vi "ResultsDB Select Column Name List.vi"() -> (0 "error out":errorcluster, 3 "FirstRow":string[](array[string]))   [LabVIEW 2021, in "SQLite.lvclass"]
doc: "开始测试时根据条目自动创建条目条目，生产文件路径。\n#2020-6-8 13:25:45"
uses:
  SQLite.lvclass
  ProcutctionStatistic.ctl
  <userlib>/_OpenG.lib/array/array.llb/Search 1D Array (String)__ogtk.vi
  SQLite.lvclass/SQLite.ctl
  <userlib>/LabSQL/LabSQL.lvlib
  vi.lib_New/TopPath/TopPath.lvlib
  <userlib>/sushu/sushu.lvlib
panel:
  out "产量统计":T1
  out "CMD":string
  out "subarray":string[](array[string])
  out "number (0 to 1)":dbl
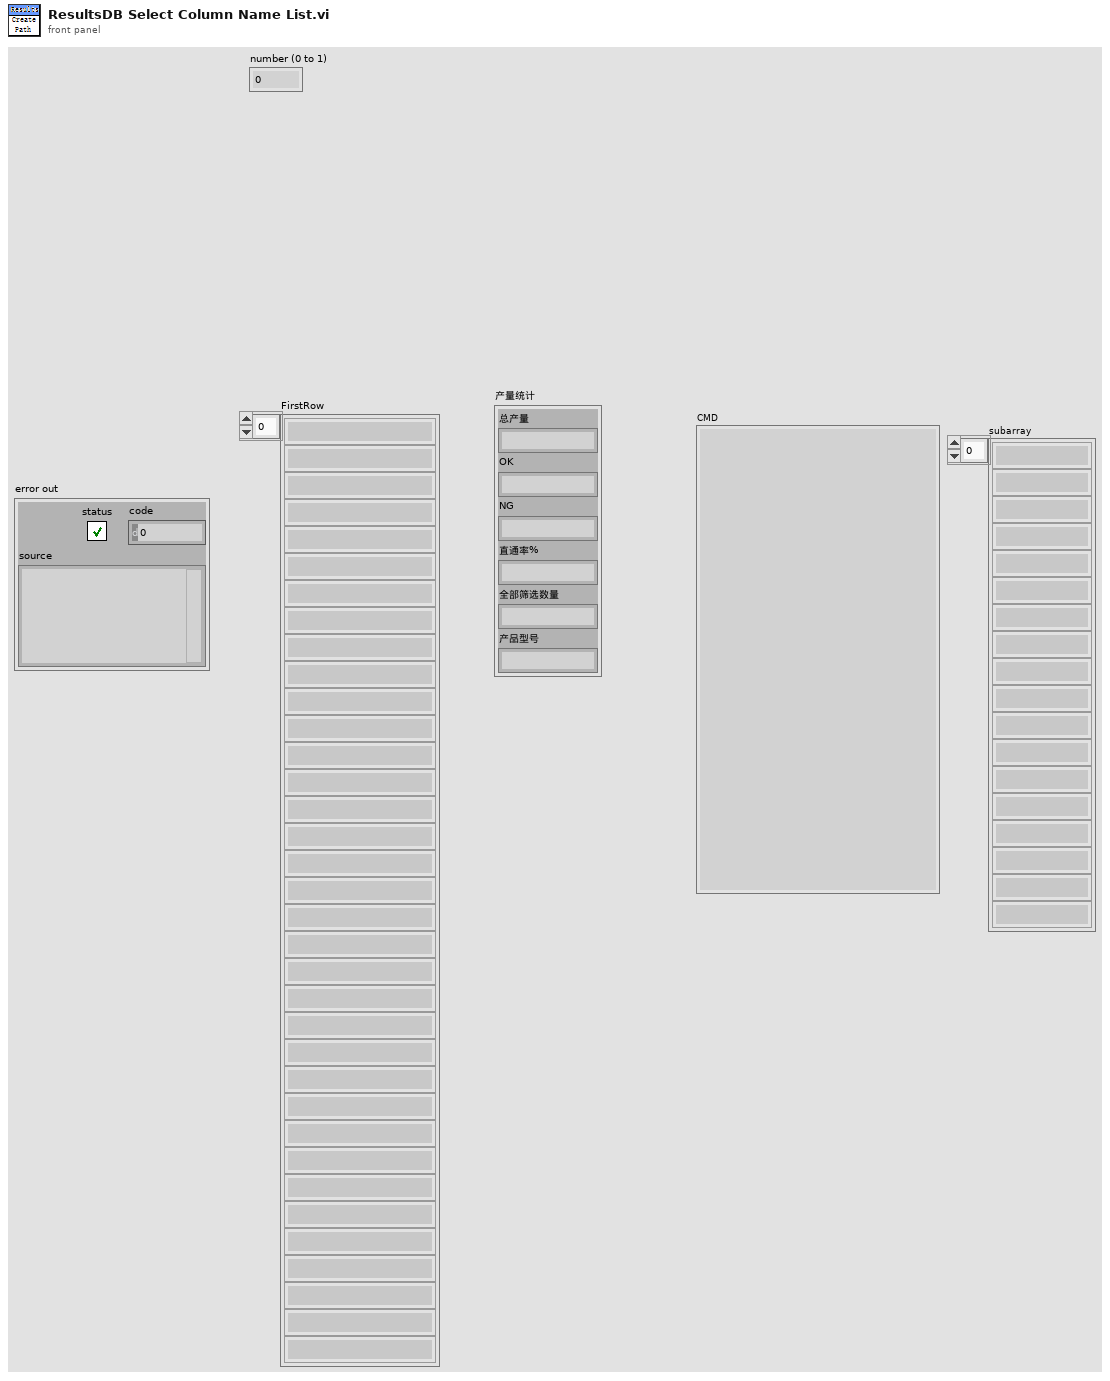
[diagram p1: front panel]
types:
  T1 = typedef "SQLite.lvclass/ProcutctionStatistic.ctl" = cluster{"总产量":string, "OK":string, "NG":string, "直通率%":string, "全部筛选数量":string, "产品型号":string}
  T2 = cluster{"Core":cluster{"Current VI Reference":refnum<vi>, "Close Panel on Exit?":bool}, "VI Name":string, "Row Numbers":string, "Update?":bool, "Results Folder path":path, "CMD":string, "RowNum":i32, "ResultFilePath":path, "InsertTimes":i32, "length":i32}
  T3 = enum16{"Other", "SQL2008", "SQLite", "Access", "MySQL"}
  T4 = typedef "TopPath.lvlib/Top Path.ctl" = cluster{"LV Source":path, "FilePath":path, "Data":path}
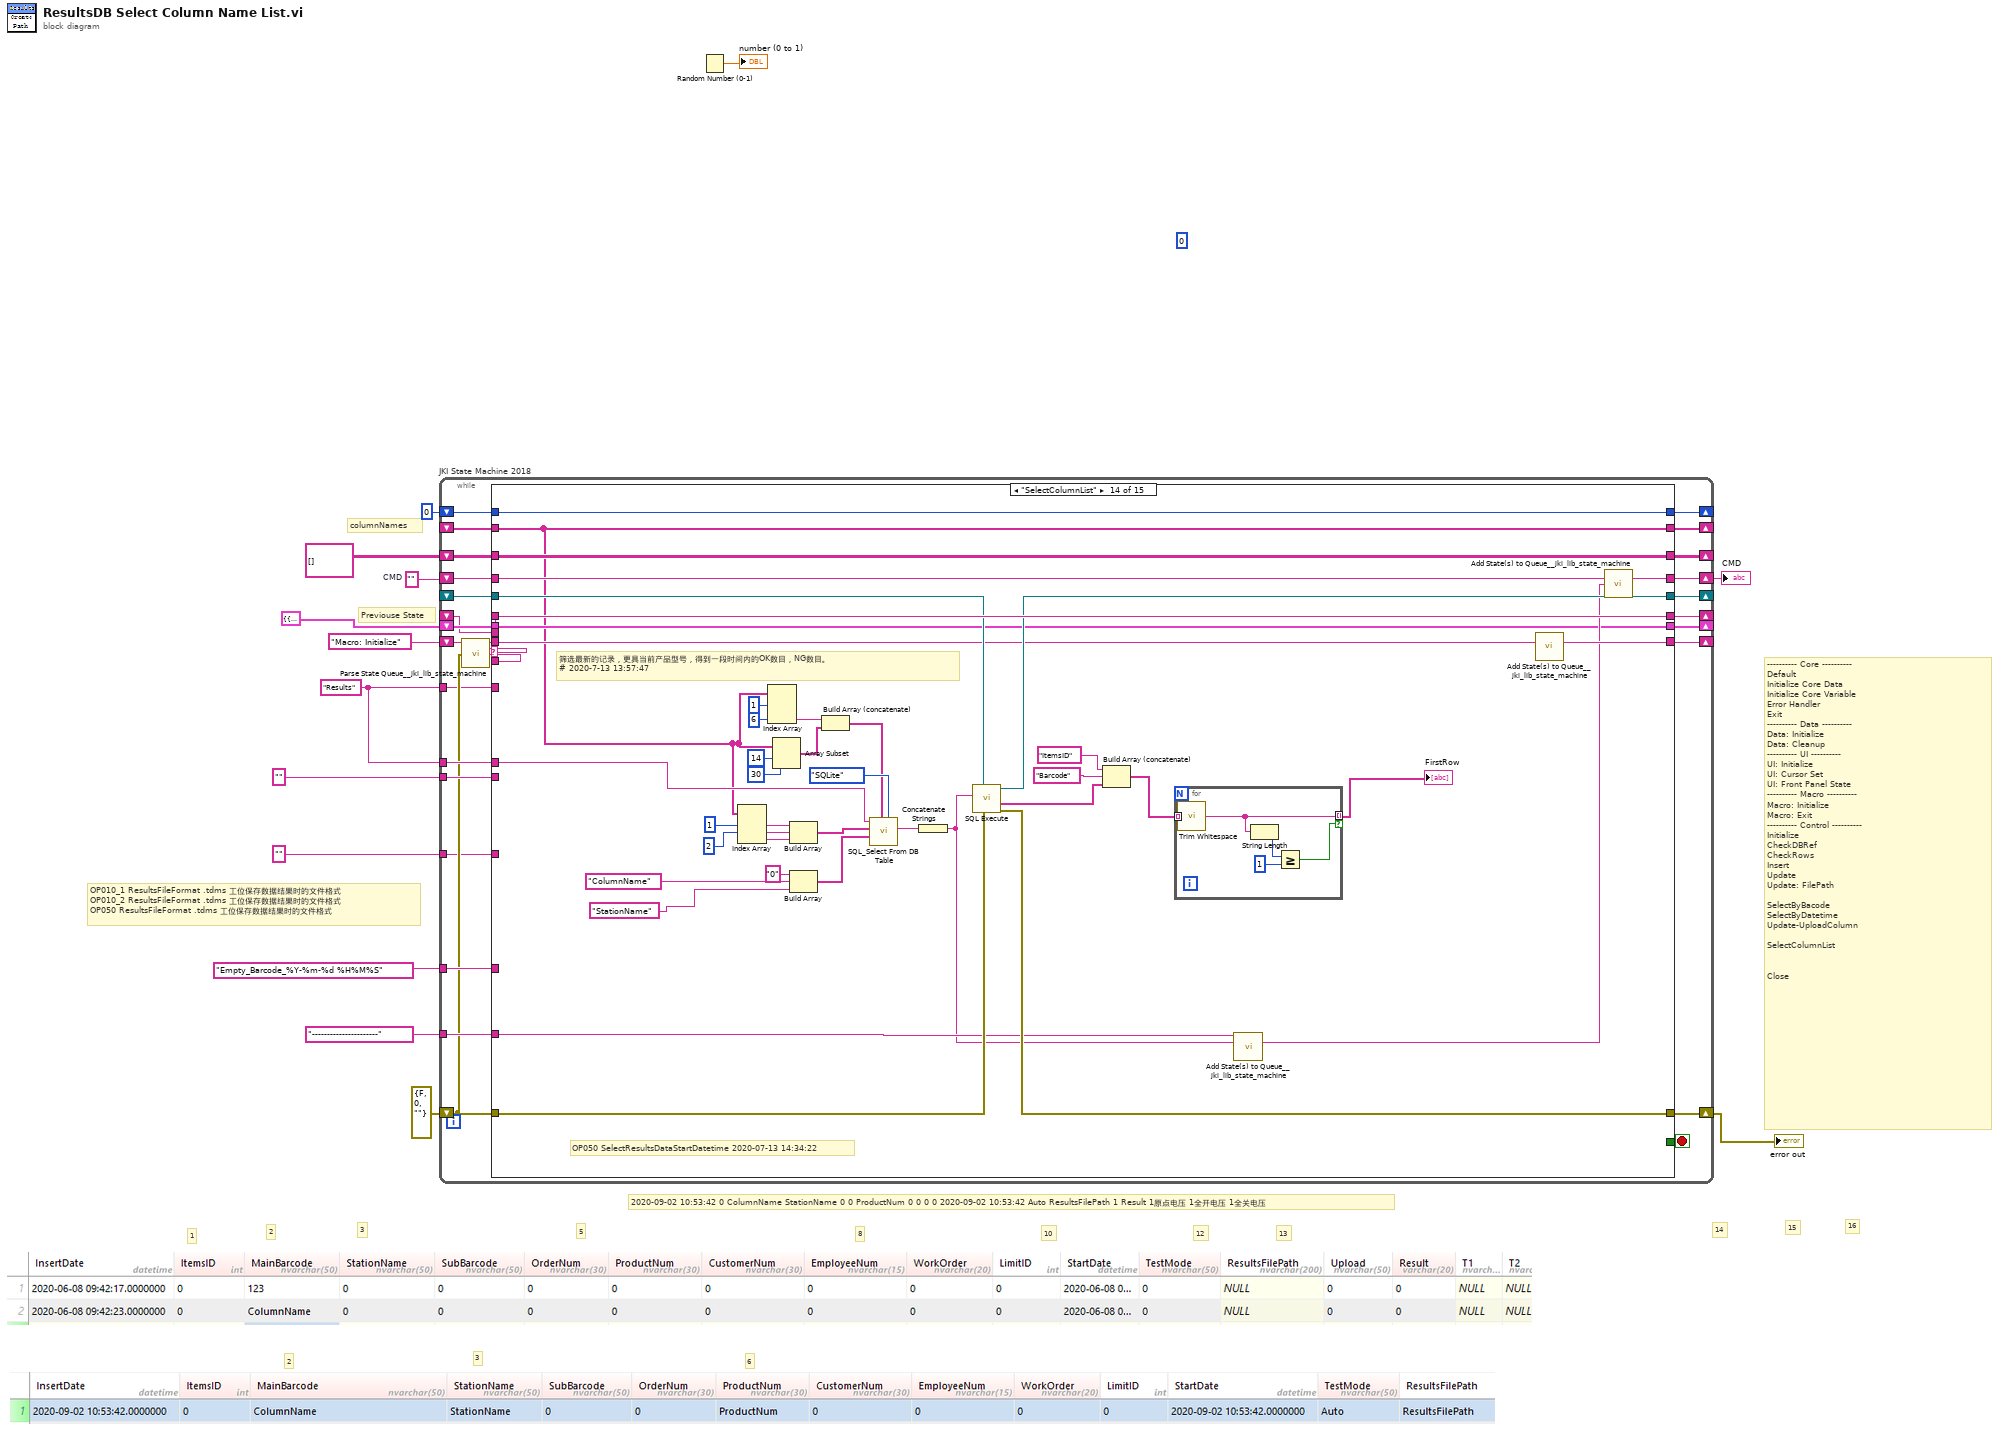
[diagram p0: block diagram]
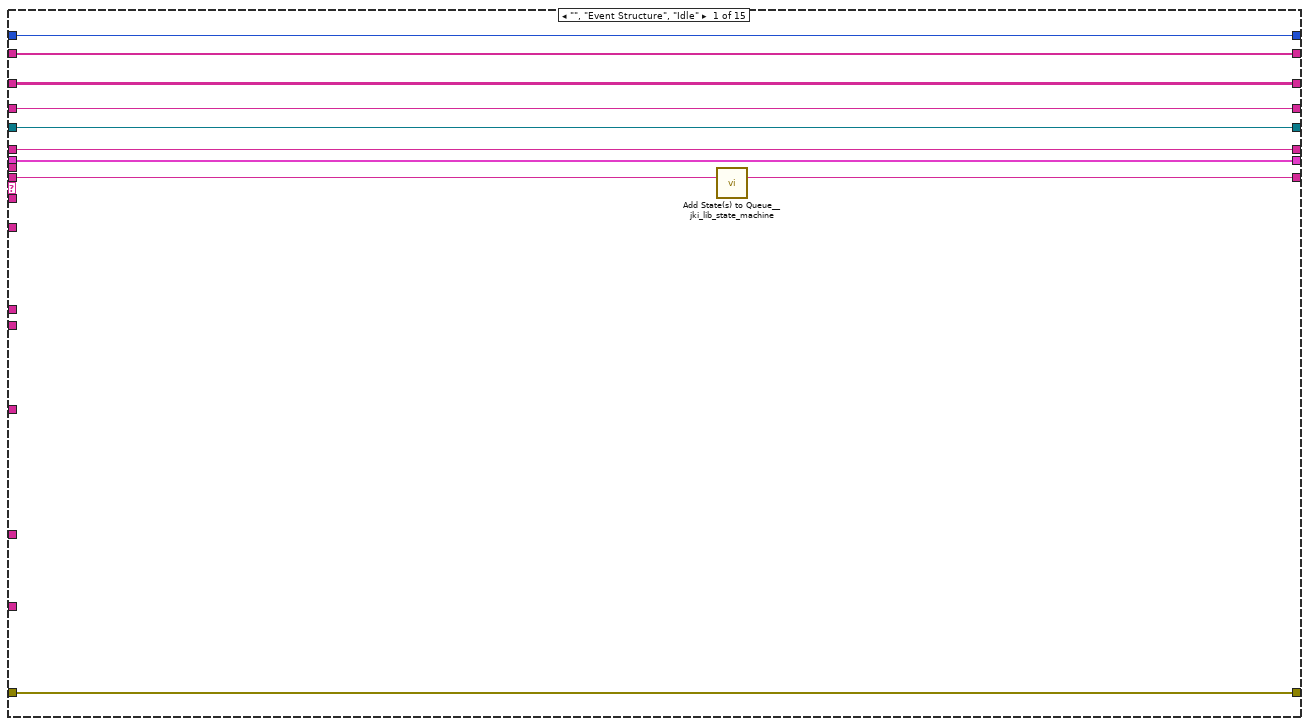
[diagram p2: hidden frame]
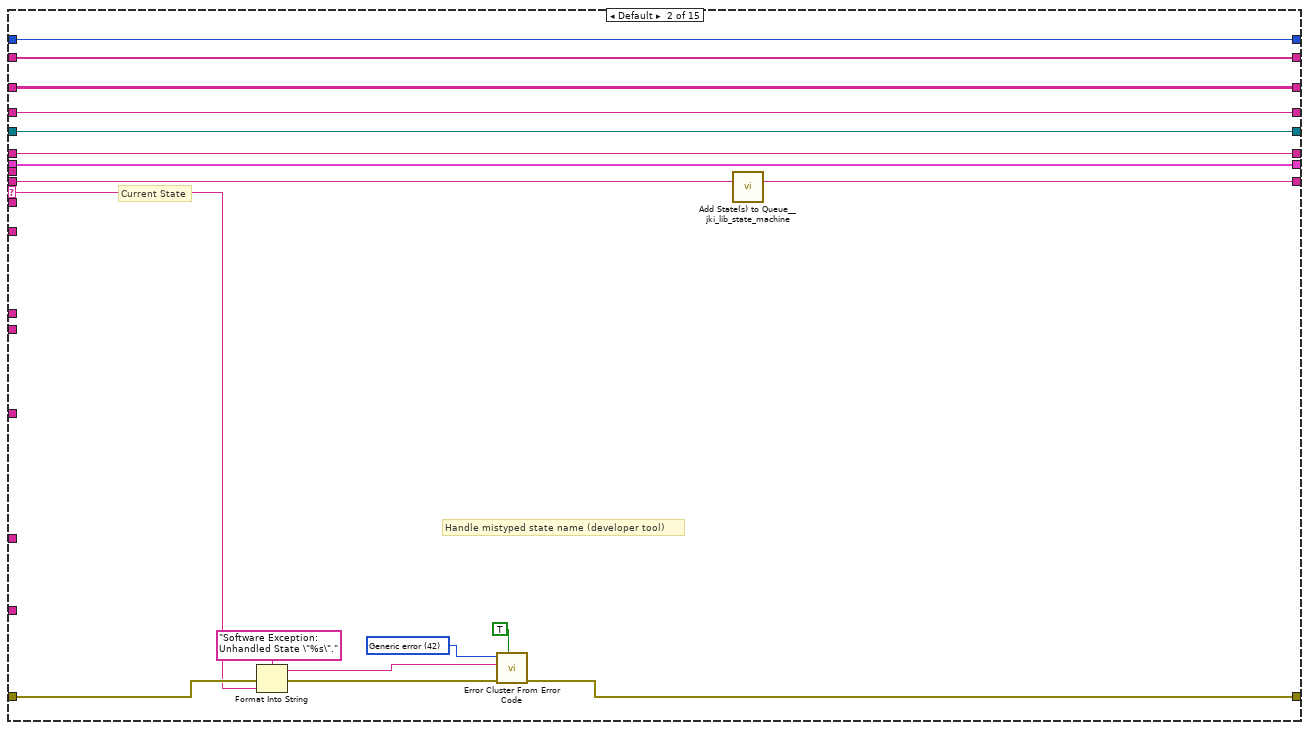
[diagram p3: hidden frame]
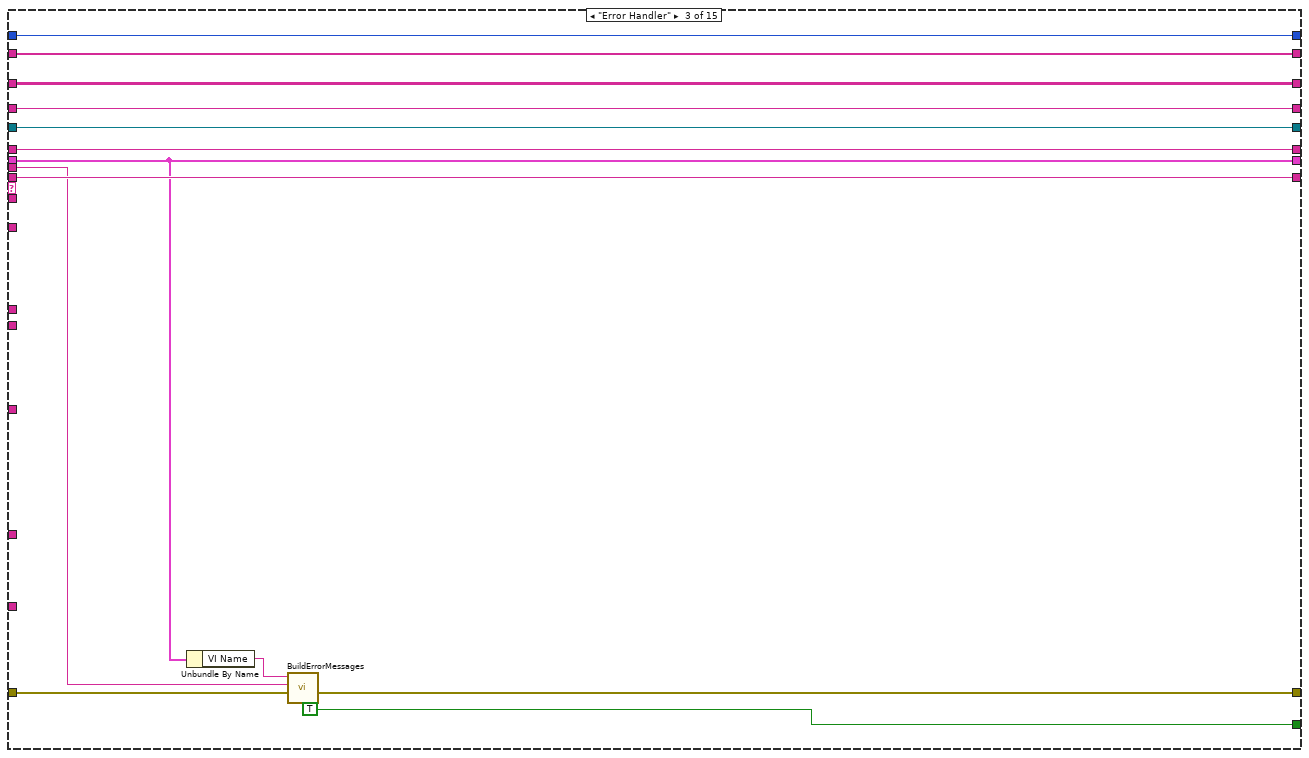
[diagram p4: hidden frame]
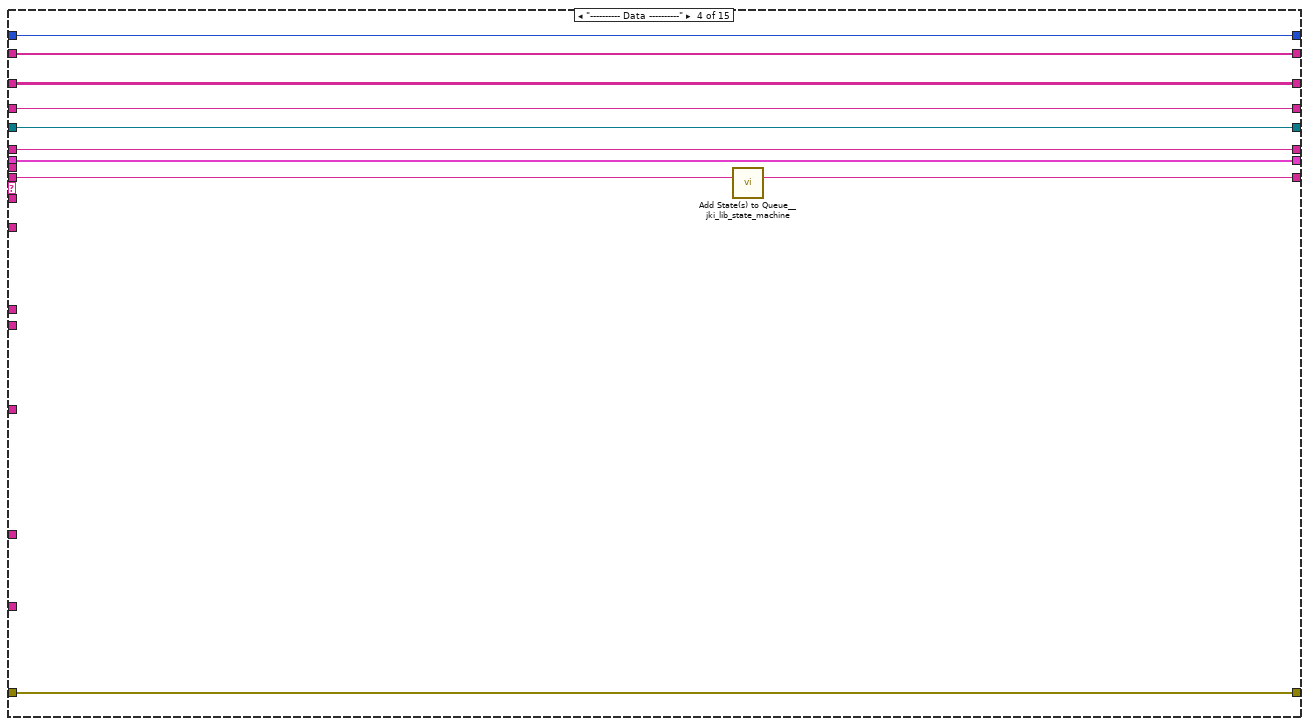
[diagram p5: hidden frame]
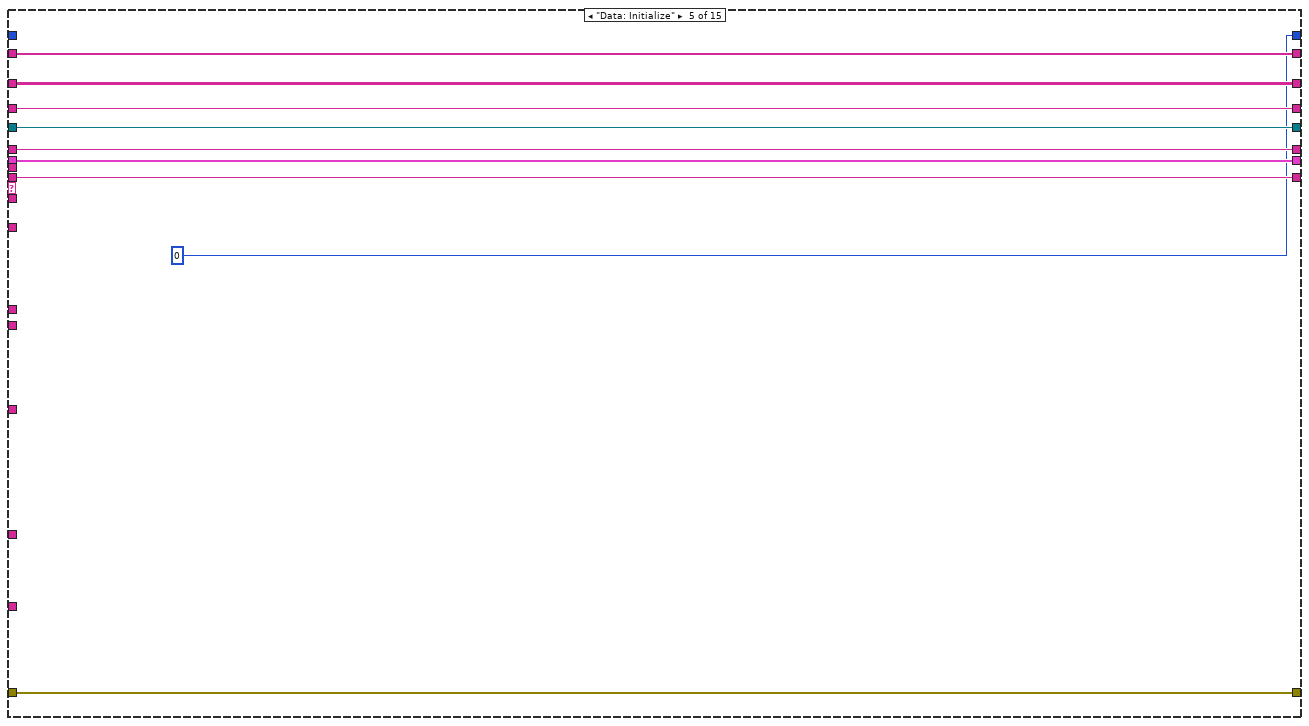
[diagram p6: hidden frame]
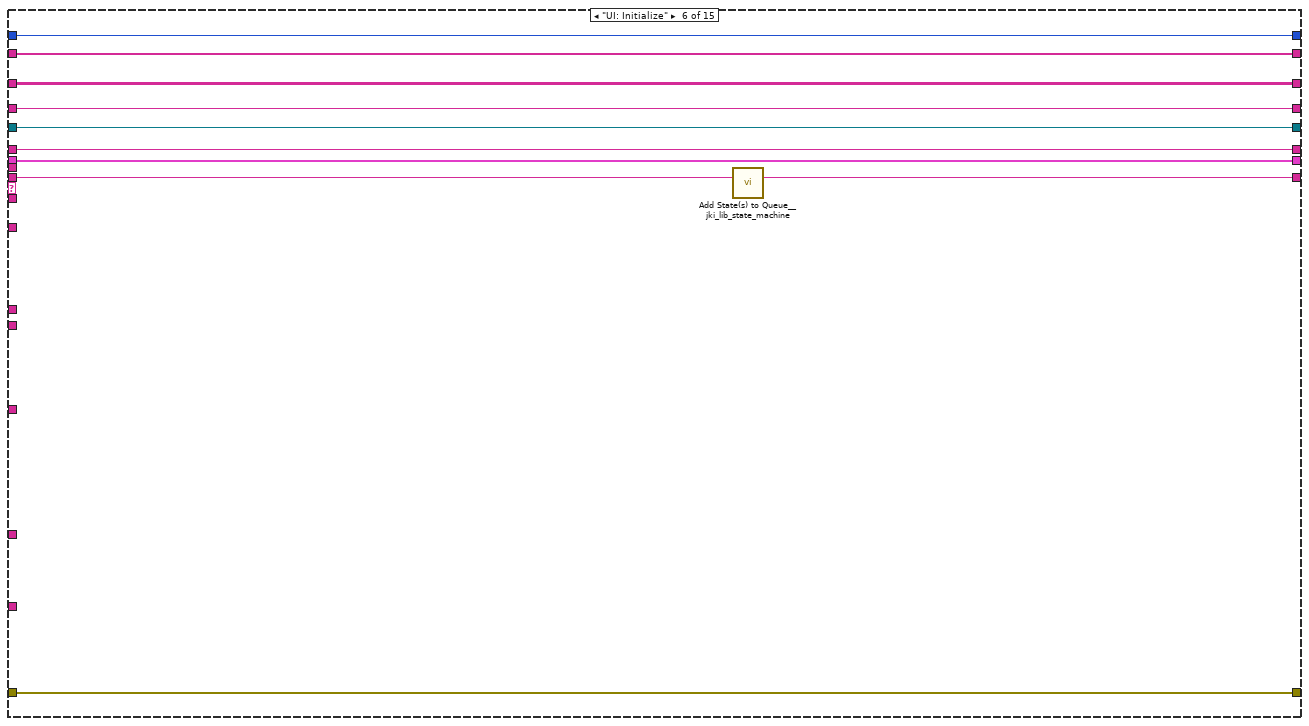
[diagram p7: hidden frame]
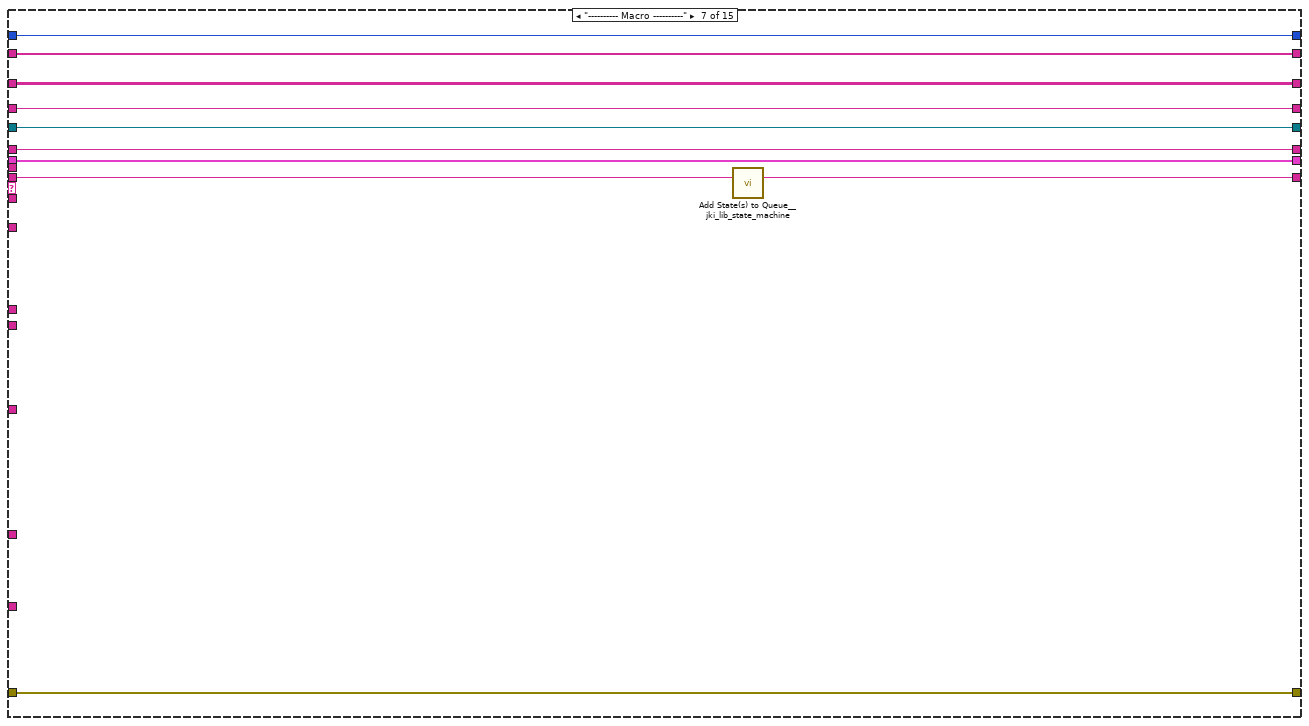
[diagram p8: hidden frame]
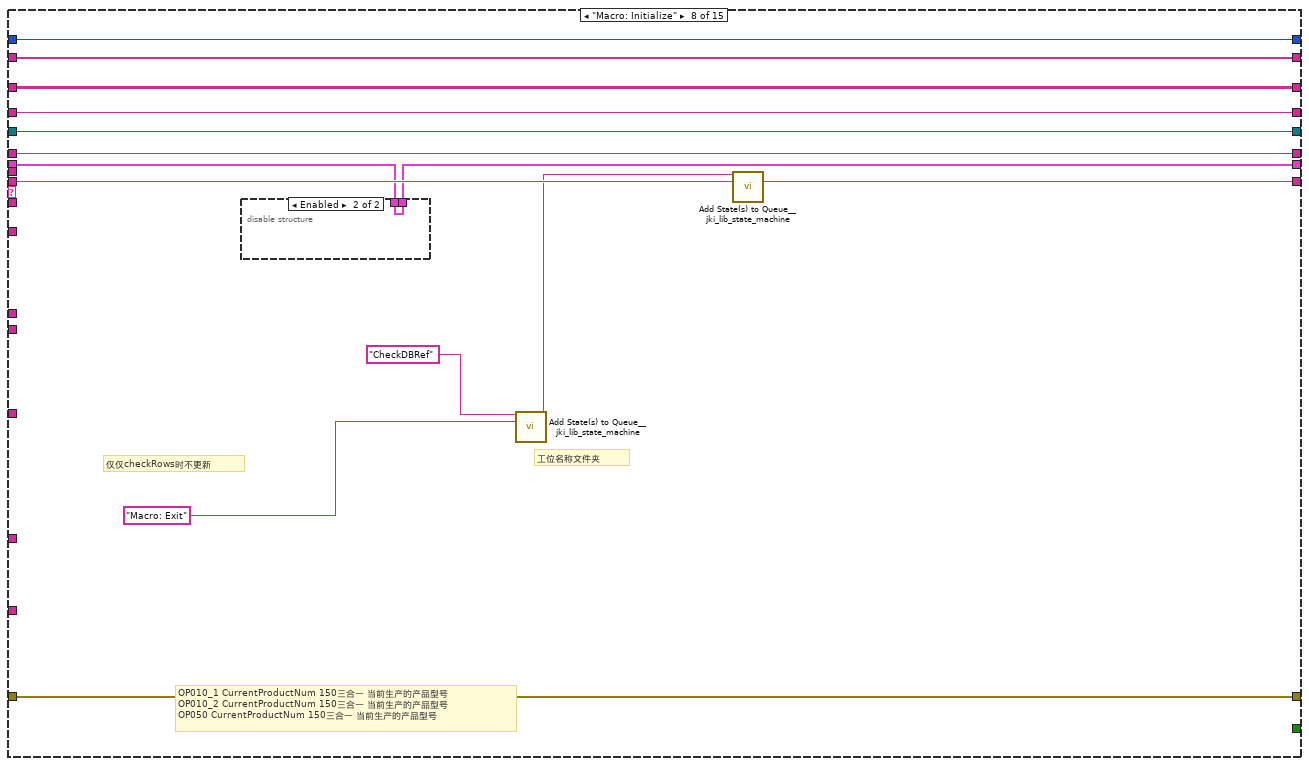
[diagram p9: hidden frame]
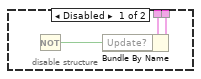
[diagram p10: hidden frame]
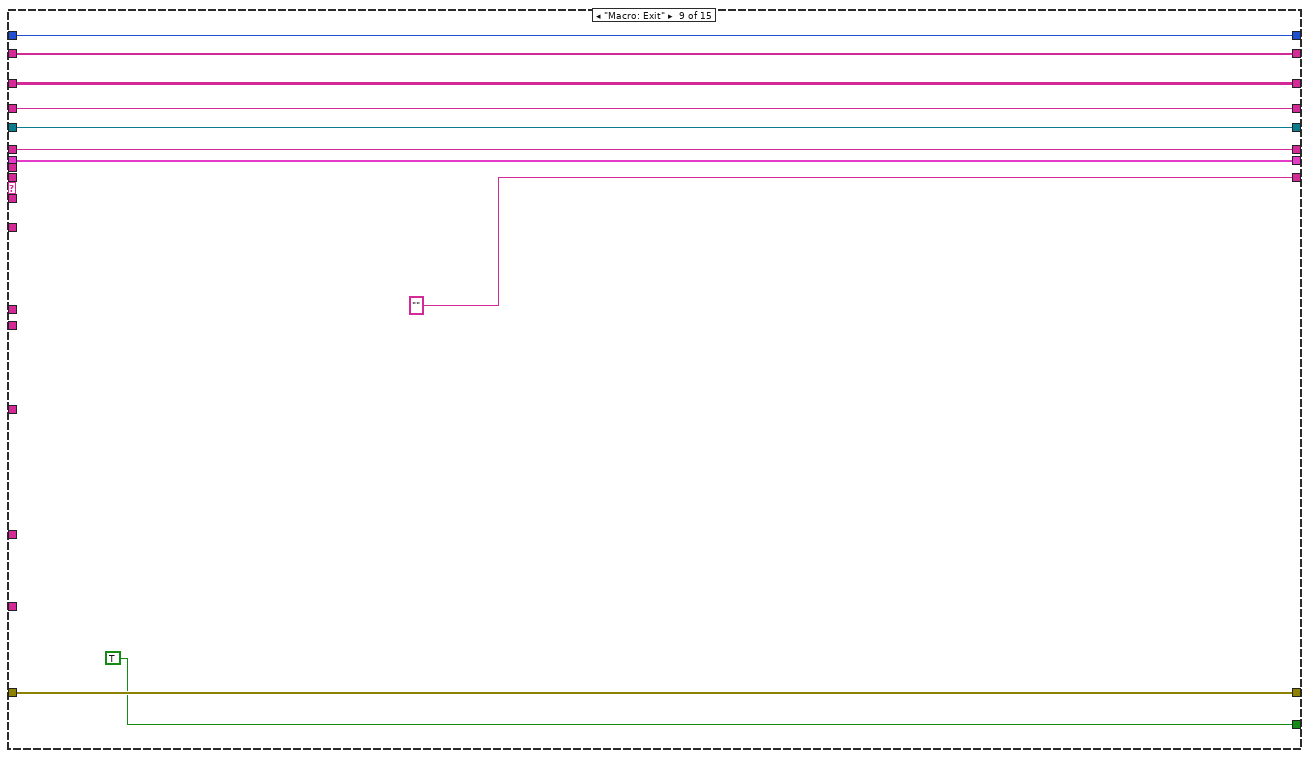
[diagram p11: hidden frame]
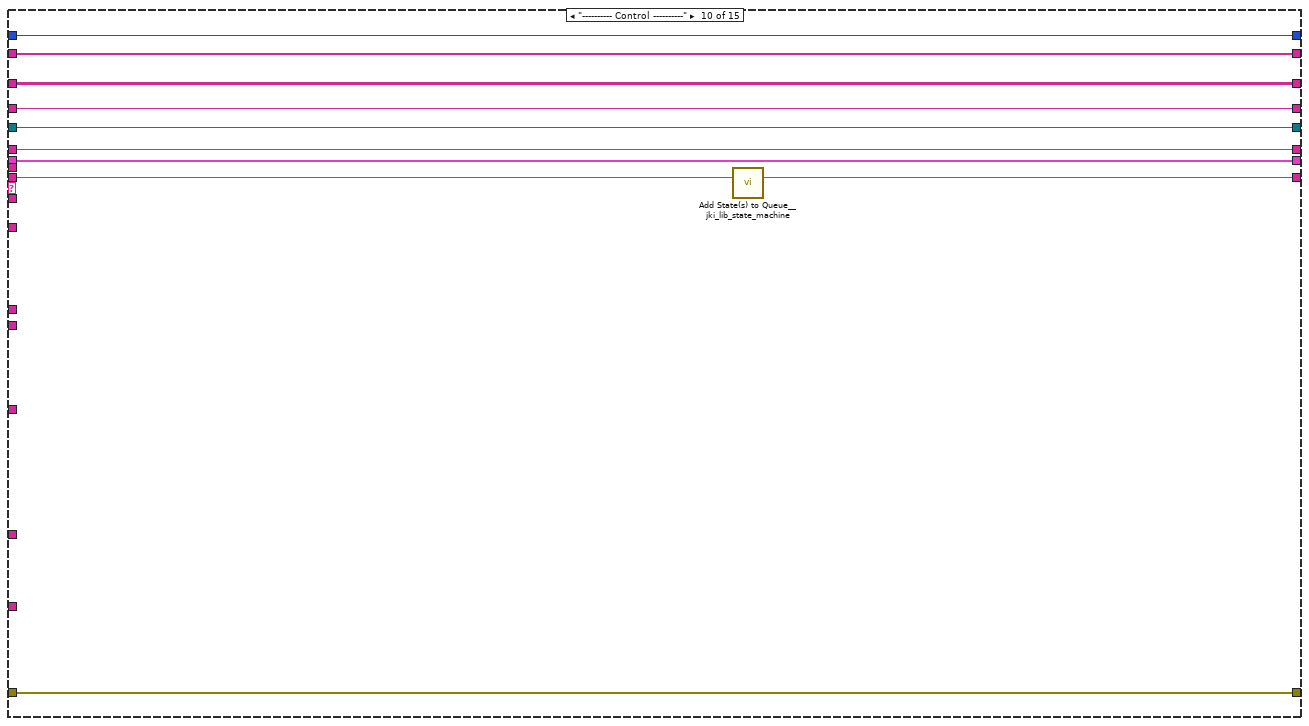
[diagram p12: hidden frame]
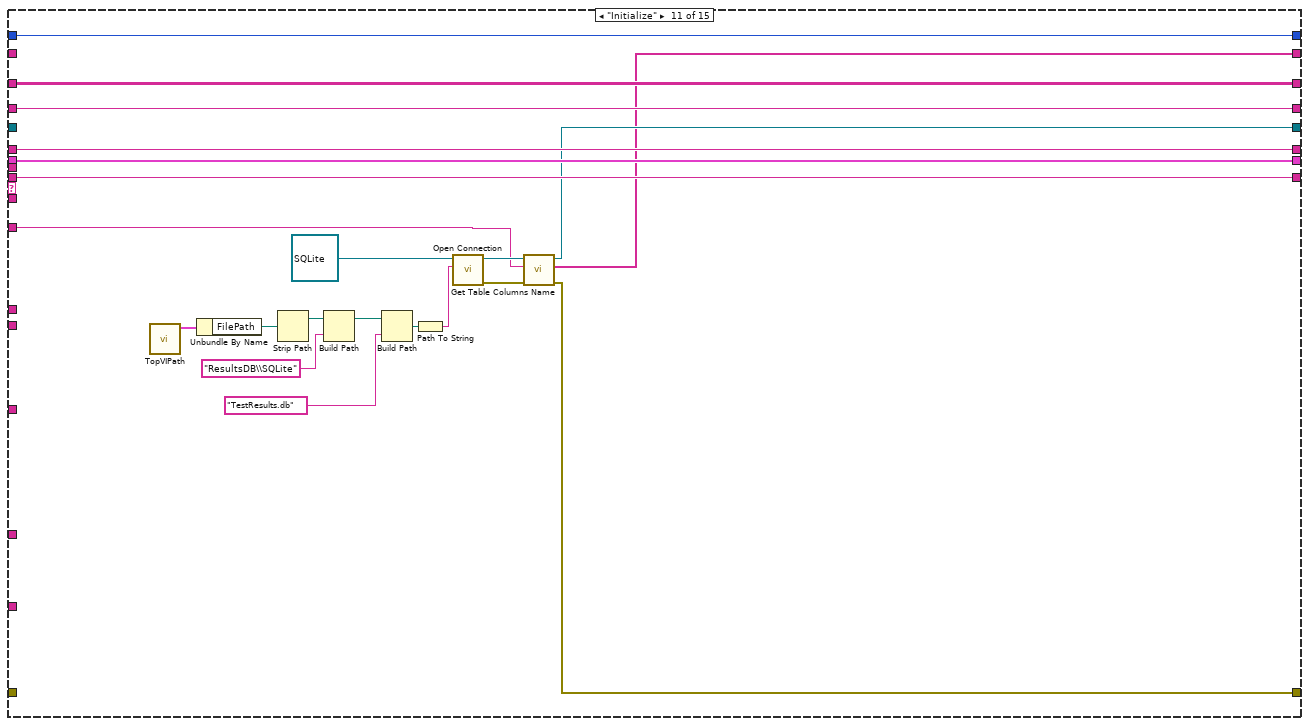
[diagram p13: hidden frame]
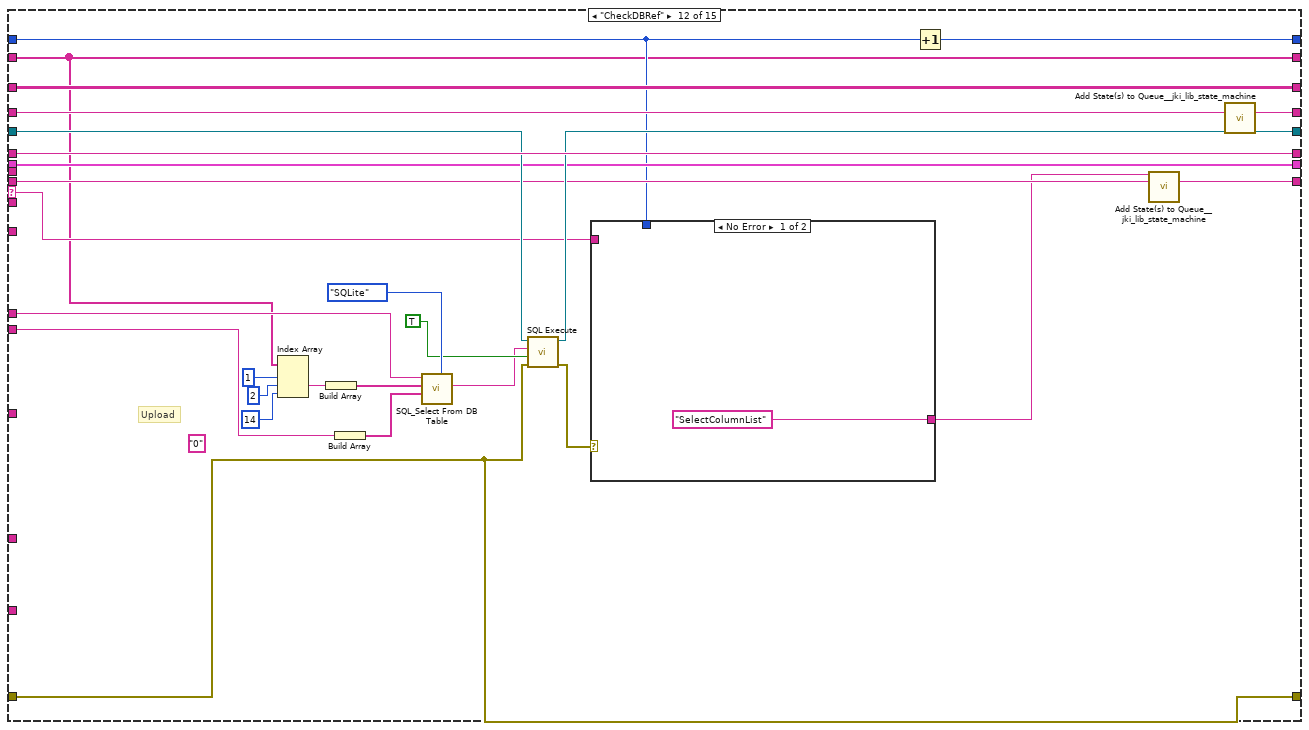
[diagram p14: hidden frame]
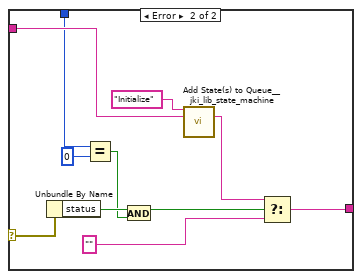
[diagram p15: hidden frame]
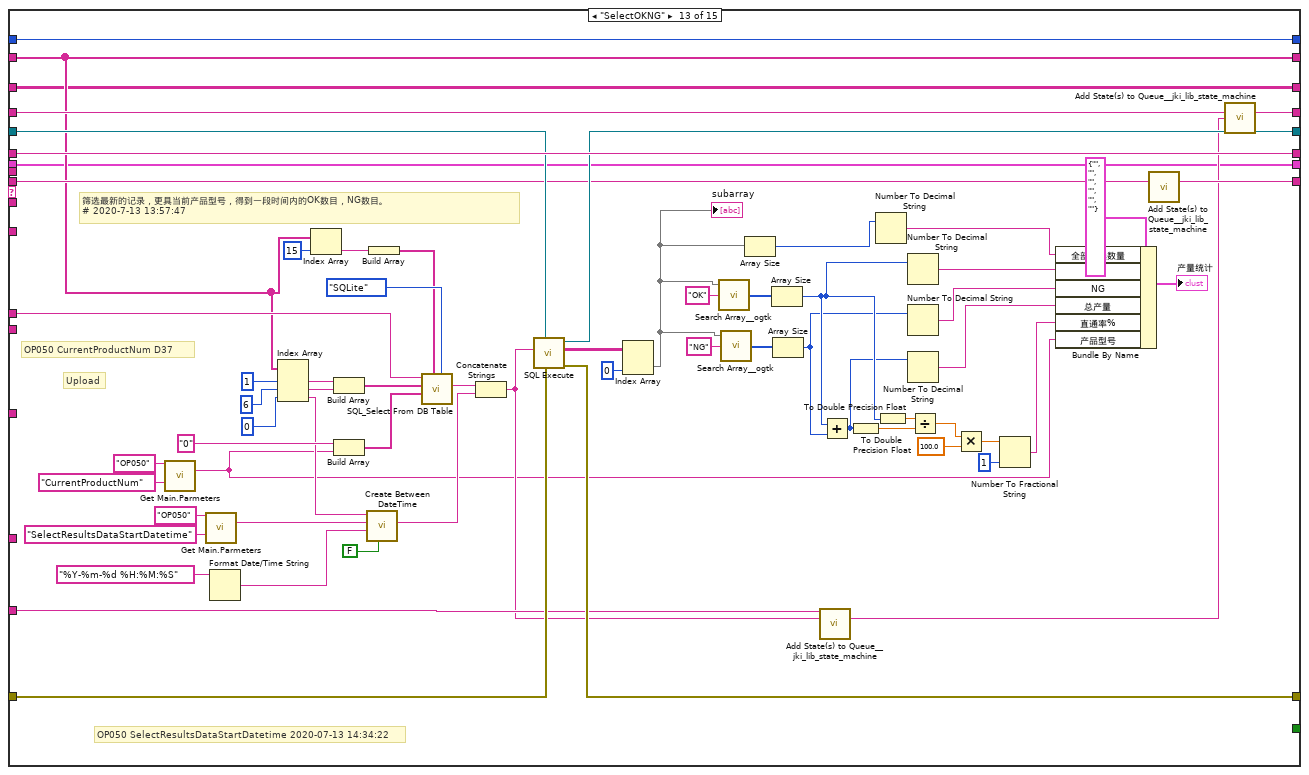
[diagram p16: hidden frame]
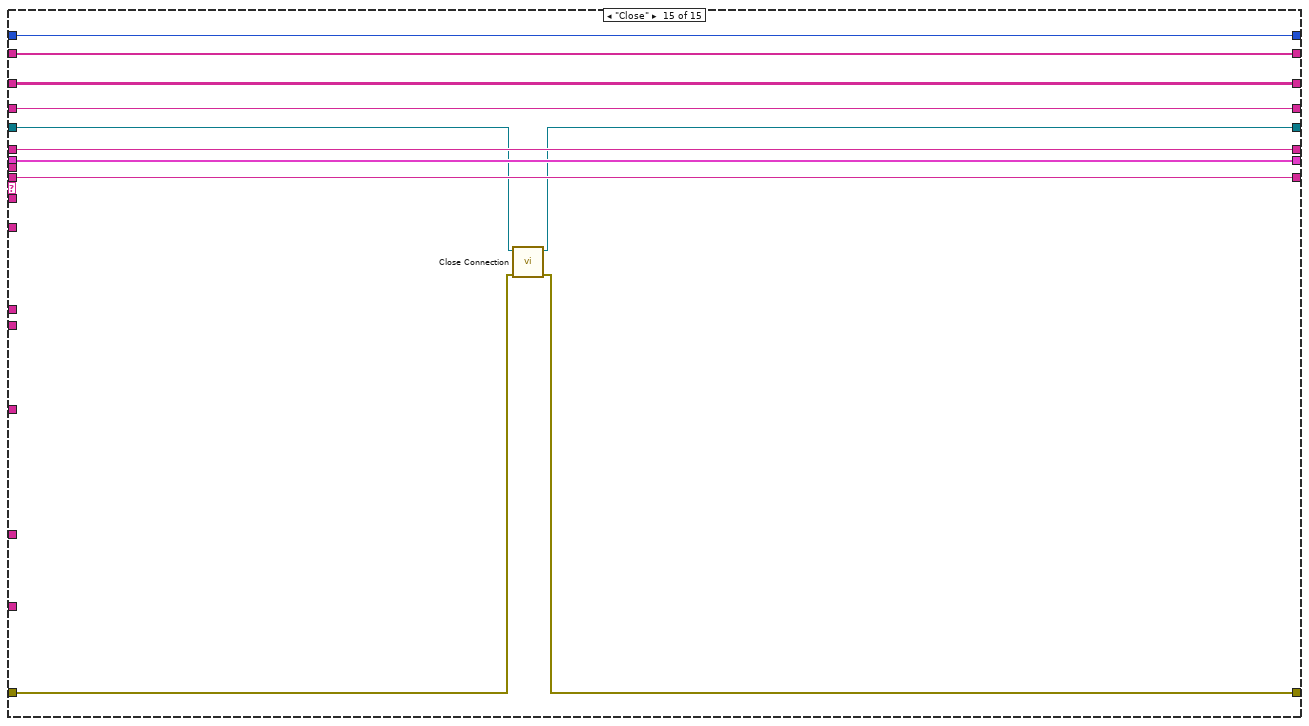
[diagram p17: hidden frame]
diagram:
  w5 = "Results" ("TableName")
  w7 = ""  # CMD
  (unwired) 0 ("index (row)")
  # "6"
  # "3"
  # "2"
  # "2020-09-02 10:53:42\t0\tColumnName\tStationName\t0\t0\tProductNum\t0\t0\t0\t0\t2020-09-02 10:53:42\tAuto\tResultsFilePath\t1\tResult\t1原点电压\t1全开电压\t1全关电压"
  # "columnNames"
  # "OP010_1\tResultsFileFormat\t.tdms\t工位保存数据结果时的文件格式\nOP010_2\tResultsFileFormat\t.tdms\t工位保存数据结果时的文件格式\nOP050\tResultsFileFormat\t.tdms\t工位保存数据结果时的文件格式"
  # "16"
  # "15"
  # "14"
  # "13"
  # "12"
  # "10"
  # "8"
  # "5"
  # "3"
  # "2"
  # "1"
  # "Previouse State"
  # "---------- Core ----------\nDefault\nInitialize Core Data\nInitialize Core Variable\nError Handler\nExit\n---------- Data ----------\nData: Initialize\nData: Cleanup\n---------- UI ----------\nUI: Initialize\nUI: Cursor Set\nUI: Front Panel State\n---------- Macro ----------\nMacro: Initialize\nMacro: Exit\n---------- Control ----------\nInitialize\nCheckDBRef\nCheckRows\nInsert\nUpdate\nUpdate: FilePath\n\nSelectByBacode\nSelectByDatetime\nUpdate-UploadColumn\n\nSelectColumnList\n\n\nClose"
  n1 = while "JKI State Machine 2018" {
    shift-right: [w36] -> _
    shift-left: T2 {"Core"={"Current VI Reference"=refnum, "Close Panel on Exit?"=FALSE}, "VI Name"="", "Row Numbers"="", "Update?"=FALSE, "Results Folder path"=path "", "CMD"="", "RowNum"=0, "ResultFilePath"=path "", "InsertTimes"=0, "length"=3} ("Data") -> [w35]
    shift-right: [w39] -> w2
    shift-left: errorcluster {"status"=FALSE, "code"=0, "source"=""} ("error out") -> [w21]
    shift-right: [w38] -> _
    shift-left: "Macro: Initialize" -> [w40]
    shift-right: [w33] -> _
    shift-left: _ -> [w34]
    shift-right: [w31] -> _
    shift-left: _ -> [w30]
    tunnel: "" ("MainBarcode") -> [w29]
    tunnel: w5 -> [w28]
    tunnel: "Empty_Barcode_%Y-%m-%d %H%M%S" ("time format string (%c)") -> [w27]
    shift-right: [w26] -> w1
    shift-left: w7 -> [w25]
    tunnel: "----------------------" ("State(s) in (\"\")") -> [w24]
    shift-right: [w22] -> _
    shift-left: string[][] [] ("Table Control") -> [w23]
    tunnel: "" ("ItemsID") -> [w20]
    tunnel: w5 -> [w19]
    shift-right: [w18] -> _
    shift-left: _ -> [w17]
    shift-right: [w15] -> _
    shift-left: 0 -> [w16]
    stop <- w37 stop-if-true
    n2 = call <vilib>:"Parse State Queue__jki_lib_state_machine.vi"("State Queue"=w40, "Error In (no error)"=w21) -> ("Remaining States"=w42:string, "Current State"=w32:string, "Arguments"=w41:string)  [unwired: 10 in, 1 out]
    n3 = case shown="\"SelectColumnList\"" w32 {
      selector: w32 -> [_ w59 _ _ _ _ _ _ _ _ _ w186 _ _ _]
      tunnel: w42 -> [w52 w63 w81 w92 w98 w111 w121 w135 _ w159 w180 w196 w274 w315 w341]
      tunnel: w41 -> [_ _ _ _ _ _ _ _ _ _ _ _ _ _ _]
      tunnel: w35 -> [w49 w61 w78 w89 w99 w109 w118 w130 w148 w156 w179 w192 w243 w299 w340]
      tunnel: [w50 w65 w74 w90 w101 w108 w119 w131 w149 w157 w163 w185 w272 w313 w331] -> w39
      tunnel: w21 -> [w50 w64 w75 w90 w101 w108 w119 w131 w149 w157 _ w185 w273 w314 w332]
      tunnel: [w51 w62 w81 w91 w98 w110 w120 w134 "" w158 w180 w197 w275 w316 w341] -> w38
      tunnel: [_ _ TRUE _ _ _ _ _ TRUE _ _ _ _ _ _] -> w37
      tunnel: [w49 w61 w78 w89 w99 w109 w118 w125 w148 w156 w179 w192 w243 w299 w340] -> w36
      tunnel: w34 -> [w48 w58 w80 w88 w100 w107 w117 w133 w147 w155 _ w200 w277 w318 w334]
      tunnel: [w48 w58 w80 w88 w100 w107 w117 w133 w147 w155 w164 w199 w276 w317 w333] -> w33
      tunnel: w32 -> [w47 w57 w79 w87 w97 w106 w116 w132 w145 w154 w178 w207 w284 w325 w339]
      tunnel: [w47 w57 w79 w87 w97 w106 w116 w132 w145 w154 w178 w207 w284 w325 w339] -> w31
      tunnel: w30 -> [_ _ w76 _ _ _ _ _ _ _ _ _ _ _ _]
      tunnel: w29 -> [_ _ _ _ _ _ _ _ _ _ _ w201 _ _ _]
      tunnel: w28 -> [_ _ _ _ _ _ _ _ _ _ _ w202 w278 w319 _]
      tunnel: w27 -> [_ _ _ _ _ _ _ _ _ _ _ _ _ _ _]
      tunnel: w25 -> [w46 w56 w73 w86 w96 w105 w115 w127 w143 w153 w177 w194 w270 w311 w338]
      tunnel: [w46 w56 w73 w86 w96 w105 w115 w127 w143 w153 w177 w195 w271 w312 w338] -> w26
      tunnel: w24 -> [_ _ _ _ _ _ _ _ _ _ _ _ w267 w308 _]
      tunnel: w23 -> [w45 w55 w72 w85 w95 w104 w114 w126 w142 w152 w176 w188 w246 w300 w337]
      tunnel: [w45 w55 w72 w85 w95 w104 w114 w126 w142 w152 w176 w188 w246 w300 w337] -> w22
      tunnel: w20 -> [_ _ _ _ _ _ _ _ _ _ _ _ _ _ _]
      tunnel: w19 -> [_ _ _ _ _ _ _ _ _ _ w162 _ _ _ _]
      tunnel: w17 -> [w44 w54 w71 w84 w94 w103 w113 w124 w141 w151 _ w181 w250 w298 w336]
      tunnel: [w44 w54 w71 w84 w94 w103 w113 w124 w141 w151 w161 w181 w250 w298 w336] -> w18
      tunnel: w16 -> [w43 w53 w70 w83 _ w102 w112 w122 w140 w150 w160 w182 w259 w304 w335]
      tunnel: [w43 w53 w70 w83 0 w102 w112 w122 w140 w150 w160 w183 w259 w304 w335] -> w15
      frame "", "Event Structure", "Idle" {
        n4 = call <vilib>:"Add State(s) to Queue__jki_lib_state_machine.vi"("State(s) in (\"\")"=w52) -> ("States Out"=w51:string)  [unwired: 14 in]
      }
      frame Default {
        w68 = 42 items=["No error", "Argument error", "Memory is full", "Out of zone", "End of file", "File already open", "Generic file I/O error", "File not found", "File permission error", "Disk is full", "Duplicate path", "Too many files open", "System feature not enabled", "Resource file not found", "Cannot add resource", "Resource not found", "Image not found", "Image memory error", "Pen does not exist", "Config type invalid", "Config token not found", "Config parse error", "Config memory error", "Bad external code format", "Bad external code offset", "External code not present", "Null window", "Destroy window error", "Null menu", "Print aborted", "Bad print record", "Print driver error", "Windows error during printing", "Memory error during printing", "Print dialog error", "Generic print error", "Invalid device refnum", "Device not found", "Device parameter error", "Device unit error", "Cannot open device", "Device call aborted", "Generic error", "Cancelled by user", "Object ID too low", "Object ID too high", "Object not in heap", "Unknown heap", "Unknown object (invalid DefProc)", "Unknown object (DefProc not in table)", "Message out of range", "Invalid (null) method", "Unknown message", "Manager call not supported", "Bad address", "Network operation in progress", "Network operation timed out", "Connection is busy", "Network attribute not supported", "Network error", "Address in use", "System out of memory", "Connection aborted", "Connection refused", "Not connected", "Already connected", "Connection closed", "Initialization error (interapplication manager)", "Bad occurrence", "Wait on unbound occurrence handler", "Occurrence queue overflow", "Datalog type conflict", "Unused", "Unrecognized type (interapplication manager)", "Memory corrupt", "Failed to make temporary DLL", "Old CIN version", "Drag socket not found", "Failed to load drop-object", "Failed to register OLE object", "Failed to release OLE object", "Format specifier type mismatch", "Unknown format specifier", "Too few format specifiers", "Too many format specifiers", "Scan failed", "Newer CIN version", "Error converting to variant", "Runtime menu error", "Password tampered", "Variant attribute not found", "Incompatible variant data type", "Event data is not available", "Event Store is not present", "Occurrence is not found", "Event Queue is not created", "Event info is not available", "Refnum passed is NULL", "Error retrieving Class GUID", "Error retrieving CoClass GUID", "Error retrieving TypeLib GUID.", "Bad built application magic bytes.", "Specific driver is different from the specific driver associated with the Logical Name.", "There is no session opened to the class driver.", "Max Error", "MAX - Error with config objects", "MAX - Error loading configuration", "MAX - Group not supported"]
        # "Current State"
        # "Handle mistyped state name (developer tool)"
        n5 = Format Into String(format string="Software Exception: Unhandled State \"%s\"." ("message"), error in=w64, w59) -> (resulting string=w67:string, error out=w66:errorcluster)  [unwired: 1 in]
        n6 = call <vilib>:"Error Cluster From Error Code.vi"("show call chain? (False)"=TRUE, "error in (no error)"=w66, "error message (\"\")"=w67, "error code (0)"=w68) -> ("error out"=w65:errorcluster)  [unwired: 5 in]
        n7 = call <vilib>:"Add State(s) to Queue__jki_lib_state_machine.vi"("State(s) in (\"\")"=w63) -> ("States Out"=w62:string)  [unwired: 14 in]
      }
      frame "Error Handler" {
        n8 = Unbundle By Name(w78) -> ("VI Name"=w77:string)
        n9 = call <userlib>:"BuildErrorMessages.vi"("error in"=w75, "ErrorCase"=w76, "VI Name"=w77) -> ("error out (no error)"=w74:errorcluster)  [unwired: 6 in, 2 out]
      }
      frame "---------- Data ----------" {
        n10 = call <vilib>:"Add State(s) to Queue__jki_lib_state_machine.vi"("State(s) in (\"\")"=w92) -> ("States Out"=w91:string)  [unwired: 14 in]
      }
      frame "Data: Initialize" {
      }
      frame "UI: Initialize" {
        n11 = call <vilib>:"Add State(s) to Queue__jki_lib_state_machine.vi"("State(s) in (\"\")"=w111) -> ("States Out"=w110:string)  [unwired: 14 in]
      }
      frame "---------- Macro ----------" {
        n12 = call <vilib>:"Add State(s) to Queue__jki_lib_state_machine.vi"("State(s) in (\"\")"=w121) -> ("States Out"=w120:string)  [unwired: 14 in]
      }
      frame "Macro: Initialize" {
        # "OP010_1\tCurrentProductNum\t150三合一\t当前生产的产品型号\nOP010_2\tCurrentProductNum\t150三合一\t当前生产的产品型号\nOP050\tCurrentProductNum\t150三合一\t当前生产的产品型号"
        # "工位名称文件夹"
        # "仅仅checkRows时不更新"
        n13 = disable-structure shown="Enabled" {
          disable-tunnel: w130 -> [w138 w139]
          disable-tunnel: [w137 w139] -> w125
          frame Disabled {
            n14 = Not() -> (.not. x?=w136:bool)  [unwired: 1 in]
            n15 = Bundle By Name(cluster=w138, "Update?"=w136) -> (w137:T2)
          }
          frame Enabled {
          }
        }
        n16 = call <vilib>:"Add State(s) to Queue__jki_lib_state_machine.vi"("State(s) in Front (\"\")"="CheckDBRef" ("State(s) in Front (\"\")"), "State(s) in (\"\")"="Macro: Exit") -> ("States Out"=w129:string)  [unwired: 13 in]
        n17 = call <vilib>:"Add State(s) to Queue__jki_lib_state_machine.vi"("State(s) in Front (\"\")"=w129, "State(s) in (\"\")"=w135) -> ("States Out"=w134:string)  [unwired: 13 in]
      }
      frame "Macro: Exit" {
      }
      frame "---------- Control ----------" {
        n18 = call <vilib>:"Add State(s) to Queue__jki_lib_state_machine.vi"("State(s) in (\"\")"=w159) -> ("States Out"=w158:string)  [unwired: 14 in]
      }
      frame "Initialize" {
        n19 = call "TopVIPath.vi"() -> ("TopPath"=w175:T4)  [unwired: 10 in, 1 out]
        n20 = Unbundle By Name(w175) -> ("FilePath"=w165:path)
        n21 = Strip Path(path=w165) -> (stripped path=w166:path)  [unwired: 1 out]
        n22 = Build Path(base path=w166, name or relative path="ResultsDB\\SQLite") -> (appended path=w168:path)
        n23 = Build Path(base path=w168, name or relative path="TestResults.db") -> (appended path=w170:path)
        n24 = Path To String(path=w170) -> (string=w171:string)
        n25 = call-dynamic "Open Connection.vi"("ConnectionString"=w171, "HostDB in"=refnum<class "SQLite.lvclass"> refnum ("SQLite.lvclass")) -> ("error out"=w173:errorcluster, "HostDB out"=w172:refnum<class "SQLite.lvclass">)  [unwired: 8 in]
        n26 = call-dynamic "Get Table Columns Name.vi"("error in (no error)"=w173, "TableName"=w162, "HostDB in"=w172) -> ("error out"=w163:errorcluster, "Table_ColunmsList"=w161:string[], "HostDB out"=w164:refnum<class "SQLite.lvclass">)  [unwired: 4 in, 2 out]
      }
      frame "CheckDBRef" {
        (unwired) "0" ("State(s) in (\"\")")
        # "Upload"
        n27 = Index Array(array=w181, index #1=1 ("index"), index #2=2 ("index"), index #3=14 ("index")) -> (element #2=w190:string)  [unwired: 2 out]
        n28 = Build Array(w190) -> (w205:string[])
        n29 = Build Array(w201) -> (w204:string[])
        n30 = call <userlib>:"SQL_Select From DB Table.vi"("DB Type"=T3."SQLite", "ColumnsValue"=w204, "ColumnsNameList"=w205, "TableName"=w202) -> ("Select SQL CMD"=w193:string)  [unwired: 7 in]
        n31 = call-dynamic "SQL Execute.vi"("error in (no error)"=w185, "Return Data (T)"=TRUE, "Command Text"=w193, "HostDB in"=w200) -> ("error out"=w187:errorcluster, "HostDB out"=w199:refnum<class "SQLite.lvclass">)  [unwired: 3 in, 3 out]
        n32 = case shown="No Error" w187 {
          selector: w187 -> [_ w215]
          tunnel: w186 -> [_ w216]
          tunnel: ["SelectColumnList" ("resulting string") w214] -> w184
          tunnel: w182 -> [_ w211]
          frame No Error {
          }
          frame Error {
            n33 = Unbundle By Name(w215) -> ("status"=w213:bool)
            n34 = Equal?(x=w211, y=0) -> (x = y?=w209:bool)
            n35 = And(x=w213, y=w209) -> (x .and. y?=w212:bool)
            n36 = call <vilib>:"Add State(s) to Queue__jki_lib_state_machine.vi"("State(s) in Front (\"\")"="Initialize" ("Remaining States"), "State(s) in (\"\")"=w216) -> ("States Out"=w217:string)  [unwired: 13 in]
            n37 = Select(t=w217, s=w212, f="") -> (s? t:f=w214:string)
          }
        }
        n38 = Increment(x=w182) -> (x+1=w183:i32)
        n39 = call <vilib>:"Add State(s) to Queue__jki_lib_state_machine.vi"("State(s) in Front (\"\")"=w184, "State(s) in (\"\")"=w196) -> ("States Out"=w197:string)  [unwired: 13 in]
        n40 = call <vilib>:"Add State(s) to Queue__jki_lib_state_machine.vi"("State(s) in (\"\")"=w194) -> ("States Out"=w195:string)  [unwired: 14 in]
      }
      frame "SelectOKNG" {
        # "OP050\tSelectResultsDataStartDatetime\t2020-07-13 14:34:22"
        # "OP050\tCurrentProductNum\tD37"
        # "筛选最新的记录，更具当前产品型号，得到一段时间内的OK数目，NG数目。\n# 2020-7-13 13:57:47"
        # "Upload"
        n41 = call "Get Main.Parmeters.vi"("Main"="OP050", "VariableName"="CurrentProductNum") -> ("Value"=w220:string)  [unwired: 6 in, 7 out]
        n42 = call "Get Main.Parmeters.vi"("Main"="OP050", "VariableName"="SelectResultsDataStartDatetime") -> ("Value"=w251:string)  [unwired: 6 in, 7 out]
        n43 = Format Date/Time String(time format string (%c)="%Y-%m-%d %H:%M:%S") -> (date/time string=w264:string)  [unwired: 2 in]
        n44 = Index Array(array=w250, index #1=1 ("index"), index #2=6 ("index"), index #3=0 ("index")) -> (element #1=w283:string, element #2=w256:string, element #3=w254:string)
        n45 = Index Array(array=w250, index=15) -> (element=w248:string)
        n46 = Build Array(w283, w256) -> (w281:string[])
        n47 = Build Array("0" ("State(s) in (\"\")"), w220) -> (w280:string[])
        n48 = call <userlib>:"Create Between DateTime.vi"("HaveWhere?"=FALSE, "End DateTime"=w264, "Start DateTime"=w251, "Column Name"=w254) -> ("Between DateTime"=w260:string)  [unwired: 7 in]
        n49 = Build Array(w248) -> (w247:string[])
        n50 = call <userlib>:"SQL_Select From DB Table.vi"("DB Type"=T3."SQLite", "SelectedColumnsNameList"=w247, "ColumnsValue"=w280, "ColumnsNameList"=w281, "TableName"=w278) -> ("Select SQL CMD"=w268:string)  [unwired: 6 in]
        n51 = Concatenate Strings(w268, w260) -> (w261:string)
        n52 = call-dynamic "SQL Execute.vi"("error in (no error)"=w273, "Command Text"=w261, "HostDB in"=w277) -> ("error out"=w272:errorcluster, "Table Control"=w245:string[][], "HostDB out"=w276:refnum<class "SQLite.lvclass">)  [unwired: 4 in, 2 out]
        n53 = Index Array(array=w245, index (col)=0 ("disabled index (col)")) -> (element=w223:string[])  [unwired: 1 in]
        "subarray" <- w223
        n54 = call-poly <userlib>:"Search Array__ogtk.vi"("Array"=w223, "Element Data"="OK") -> ("Indices of Elements"=w240:i32[])  [unwired: 7 in]
        n55 = call-poly <userlib>:"Search Array__ogtk.vi"("Array"=w223, "Element Data"="NG") -> ("Indices of Elements"=w239:i32[])  [unwired: 7 in]
        n56 = Array Size(array=w223) -> (size(s)=w221:i32)
        n57 = Array Size(array=w240) -> (size(s)=w234:i32)
        n58 = Array Size(array=w239) -> (size(s)=w233:i32)
        n59 = call <vilib>:"Add State(s) to Queue__jki_lib_state_machine.vi"("State(s) in Front (\"\")"=w267, "State(s) in (\"\")"=w261) -> ("States Out"=w269:string)  [unwired: 13 in]
        n60 = Add(x=w234, y=w233) -> (x+y=w232:i32)
        n61 = To Double Precision Float(number=w232) -> (double precision float=w237:dbl)
        n62 = Number To Decimal String(number=w221) -> (decimal integer string=w222:string)  [unwired: 1 in]
        n63 = To Double Precision Float(number=w234) -> (double precision float=w238:dbl)
        n64 = Number To Decimal String(number=w234) -> (decimal integer string=w227:string)  [unwired: 1 in]
        n65 = Number To Decimal String(number=w233) -> (decimal integer string=w226:string)  [unwired: 1 in]
        n66 = Number To Decimal String(number=w232) -> (decimal integer string=w225:string)  [unwired: 1 in]
        n67 = Divide(x=w238, y=w237) -> (x/y=w236:dbl)
        n68 = Multiply(x=w236, y=100.0) -> (x*y=w231:dbl)
        n69 = Number To Fractional String(number=w231, precision (6)=i16 1) -> (F-format string=w224:string)  [unwired: 2 in]
        n70 = Bundle By Name(cluster=T1 {"总产量"="", "OK"="", "NG"="", "直通率%"="", "全部筛选数量"="", "产品型号"=""} ("产量统计"), "全部筛选数量"=w222, "OK"=w227, "NG"=w226, "总产量"=w225, "直通率%"=w224, "产品型号"=w220) -> (→"产量统计":T1)
        n71 = call <vilib>:"Add State(s) to Queue__jki_lib_state_machine.vi"("State(s) in (\"\")"=w274) -> ("States Out"=w275:string)  [unwired: 14 in]
        n72 = call <vilib>:"Add State(s) to Queue__jki_lib_state_machine.vi"("State(s) in (\"\")"=w270, "State(s) at Back (\"\")"=w269) -> ("States Out"=w271:string)  [unwired: 13 in]
      }
      frame "SelectColumnList" {
        # "OP050\tSelectResultsDataStartDatetime\t2020-07-13 14:34:22"
        # "筛选最新的记录，更具当前产品型号，得到一段时间内的OK数目，NG数目。\n# 2020-7-13 13:57:47"
        n73 = Index Array(array=w298, index #1=1 ("index"), index #2=2 ("index")) -> (element #1=w324:string, element #2=w303:string, element #3=w286:string)  [unwired: 1 in]
        n74 = Index Array(array=w298, index #1=1 ("index"), index #3=6 ("index")) -> (element #3=w296:string)  [unwired: 1 in, 2 out]
        n75 = Array Subset(array=w298, index=14, length=30) -> (w293:string[])
        n76 = Build Array(w324, w303, w286) -> (w322:string[])
        n77 = Build Array("0" ("element"), "ColumnName" ("State(s) in (\"\")"), "StationName" ("VariableName")) -> (w321:string[])
        n78 = Build Array (concatenate)(w296, w293) -> (w301:string[])
        n79 = call <userlib>:"SQL_Select From DB Table.vi"("DB Type"=T3."SQLite", "SelectedColumnsNameList"=w301, "ColumnsValue"=w321, "ColumnsNameList"=w322, "TableName"=w319) -> ("Select SQL CMD"=w309:string)  [unwired: 6 in]
        n80 = Concatenate Strings(w309) -> (w305:string)
        n81 = call-dynamic "SQL Execute.vi"("error in (no error)"=w314, "Command Text"=w305, "HostDB in"=w318) -> ("error out"=w313:errorcluster, "FirstRow"=w290:string[], "HostDB out"=w317:refnum<class "SQLite.lvclass">)  [unwired: 4 in, 2 out]
        n82 = Build Array (concatenate)("ItemsID" ("State(s) in (\"\")"), "Barcode" ("element"), w290) -> (w289:string[])
        n83 = for {
          tunnel: w289 -> [w330] mode=indexing
          tunnel: [w327] -> w288 mode=indexing if=w326
          n84 = call <vilib>:"Trim Whitespace.vi"("string"=w330) -> ("trimmed string"=w327:string)  [unwired: 1 in]
          n85 = String Length(string=w327) -> (length=w329:i32)
          n86 = Greater Or Equal?(x=w329, y=1) -> (x >= y?=w326:bool)
        }
        "FirstRow" <- w288
        n87 = call <vilib>:"Add State(s) to Queue__jki_lib_state_machine.vi"("State(s) in Front (\"\")"=w308, "State(s) in (\"\")"=w305) -> ("States Out"=w310:string)  [unwired: 13 in]
        n88 = call <vilib>:"Add State(s) to Queue__jki_lib_state_machine.vi"("State(s) in (\"\")"=w315) -> ("States Out"=w316:string)  [unwired: 14 in]
        n89 = call <vilib>:"Add State(s) to Queue__jki_lib_state_machine.vi"("State(s) in (\"\")"=w311, "State(s) at Back (\"\")"=w310) -> ("States Out"=w312:string)  [unwired: 13 in]
      }
      frame "Close" {
        n90 = call-dynamic "Close Connection.vi"("error in (no error)"=w332, "HostDB in"=w334) -> ("error out"=w331:errorcluster, "HostDB out"=w333:refnum<class "SQLite.lvclass">)  [unwired: 8 in]
      }
    }
  }
  "error out" <- w2
  "CMD" <- w1
  n91 = Random Number (0-1)() -> (number: 0 to 1=→"number (0 to 1)":dbl)
